vi "SessionManagementService UnregisterMultiplexerSessions.vi"(6 "contextId":T1, 8 "error in":errorcluster, 9 "timeout (ms)":i32=-1, 10 "Request Data":T3, 11 "gRPC ID":T1) -> (0 "error out":errorcluster, 2 "Response Data":T2, 3 "gRPC ID out":T1)   [LabVIEW 2020, in "ni.measurementlink.sessionmanagement.v1.api.lvlib"]
uses:
  ni.measurementlink.sessionmanagement.v1.api.lvlib
  14035477-4c25-4107-8ed5-d0c4ef420ce5.vi
  RPC Messages/ni_measurementlink_sessionmanagement_v1_UnregisterMultiplexerSessionsResponse_Flat.ctl
  <vilib>/gRPC/LabVIEW gRPC Library/Shared/grpcId.ctl
  <vilib>/gRPC/LabVIEW gRPC Library/grpc-lvsupport-release.lvlib
  RPC Messages/ni_measurementlink_sessionmanagement_v1_UnregisterMultiplexerSessionsResponse.ctl
  RPC Messages/nidevice_grpc_Session.ctl
  RPC Messages/ni_measurementlink_sessionmanagement_v1_MultiplexerSessionInformation.ctl
  RPC Messages/ni_measurementlink_sessionmanagement_v1_UnregisterMultiplexerSessionsRequest.ctl
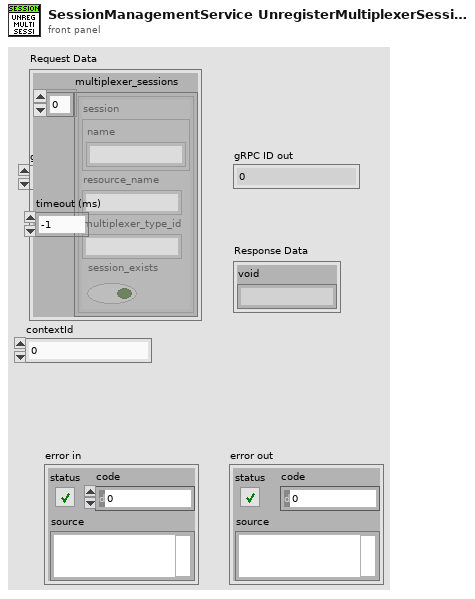
[diagram p1: front panel]
types:
  T1 = typedef "grpc-lvsupport-release.lvlib/grpcId.ctl" = u64
  T2 = typedef "ni.measurementlink.sessionmanagement.v1.api.lvlib/ni_measurementlink_sessionmanagement_v1_UnregisterMultiplexerSessionsResponse.ctl" = cluster{"void":string}
  T3 = typedef "ni.measurementlink.sessionmanagement.v1.api.lvlib/ni_measurementlink_sessionmanagement_v1_UnregisterMultiplexerSessionsRequest.ctl" = cluster{"multiplexer_sessions":T4[]}
  T4 = typedef "ni.measurementlink.sessionmanagement.v1.api.lvlib/ni_measurementlink_sessionmanagement_v1_MultiplexerSessionInformation.ctl" = cluster{"session":T5, "resource_name":string, "multiplexer_type_id":string, "session_exists":bool}
  T5 = typedef "ni.measurementlink.sessionmanagement.v1.api.lvlib/nidevice_grpc_Session.ctl" = cluster{"name":string}
  T6 = typedef "ni.measurementlink.sessionmanagement.v1.api.lvlib/ni_measurementlink_sessionmanagement_v1_UnregisterMultiplexerSessionsResponse_Flat.ctl" = cluster{"void":string}
  T7 = typedef "ni.measurementlink.sessionmanagement.v1.api.lvlib/ni_measurementlink_sessionmanagement_v1_UnregisterMultiplexerSessionsRequest_Flat.ctl" = cluster{"multiplexer_sessions":T8[]}
  T8 = typedef "ni.measurementlink.sessionmanagement.v1.api.lvlib/ni_measurementlink_sessionmanagement_v1_MultiplexerSessionInformation_Flat.ctl" = cluster{"session":T9, "resource_name":string, "multiplexer_type_id":string, "session_exists":bool}
  T9 = typedef "ni.measurementlink.sessionmanagement.v1.api.lvlib/nidevice_grpc_Session_Flat.ctl" = cluster{"name":string}
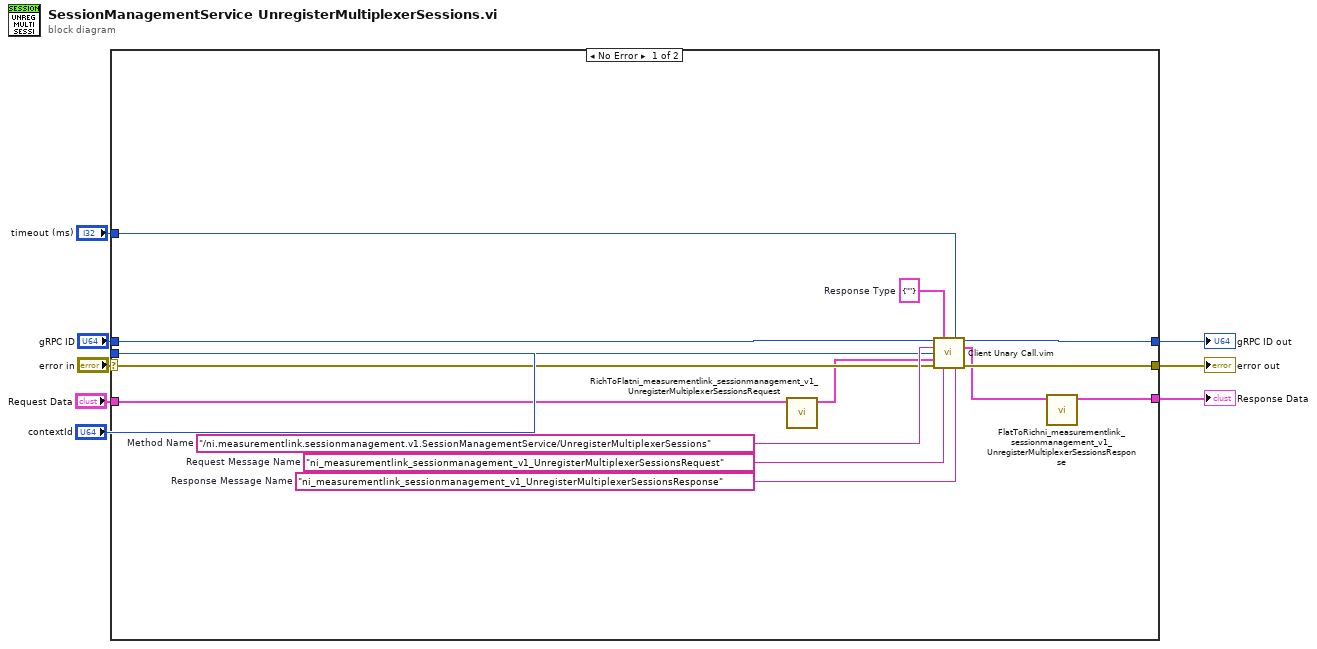
[diagram p0: block diagram]
diagram:
  n1 = case shown="No Error" "error in" {
    selector: "error in" -> [w18 w23]
    tunnel: [w17 w23] -> w7
    tunnel: "gRPC ID" -> [w16 w24]
    tunnel: [w15 w24] -> w5
    tunnel: "Request Data" -> [w12 _]
    tunnel: [w9 _] -> w3
    tunnel: "timeout (ms)" -> [w14 _]
    tunnel: "contextId" -> [w13 _]
    frame No Error {
      w19 = "ni_measurementlink_sessionmanagement_v1_UnregisterMultiplexerSessionsResponse"  # Response Message Name
      w20 = "ni_measurementlink_sessionmanagement_v1_UnregisterMultiplexerSessionsRequest"  # Request Message Name
      w21 = T6 {"void"=""}  # Response Type
      w22 = "/ni.measurementlink.sessionmanagement.v1.SessionManagementService/UnregisterMultiplexerSessions"  # Method Name
      n2 = call "RichToFlatni_measurementlink_sessionmanagement_v1_UnregisterMultiplexerSessionsRequest.vi"("InputCluster"=w12) -> ("OutputCluster"=w11:T7)  [unwired: 10 in]
      n3 = call "Client Unary Call.vim"("ClientID in"=w16, "Response Type"=w21, "timeout (ms)"=w14, "Method Name"=w22, "contextId"=w13, "Request Data"=w11, "error in"=w18, "Request Message Name"=w20, "Response Message Name"=w19) -> ("ClientID out"=w15:u64, "Response Data"=w10:T6, "error out"=w17:errorcluster)  [unwired: 4 in]
      n4 = call "FlatToRichni_measurementlink_sessionmanagement_v1_UnregisterMultiplexerSessionsResponse.vi"("InputCluster"=w10) -> ("OutputCluster"=w9:T2)  [unwired: 10 in]
    }
    frame Error {
    }
  }
  "error out" <- w7
  "gRPC ID out" <- w5
  "Response Data" <- w3
